vi "PLL.vi"(2 "Local Oscillator":waveform(dbl), 3 "Input Waveform":waveform(dbl)) -> (0 "Phase Difference":dbl)   [LabVIEW 2014]
uses:
  <vilib>/Analysis/NI_AALPro.lvlib
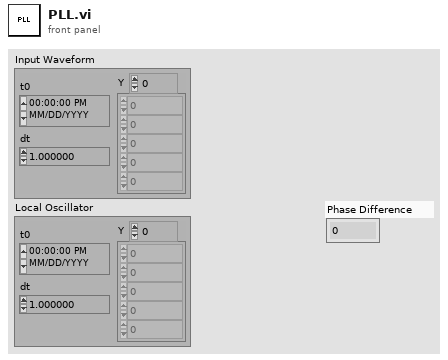
[diagram p1: front panel]
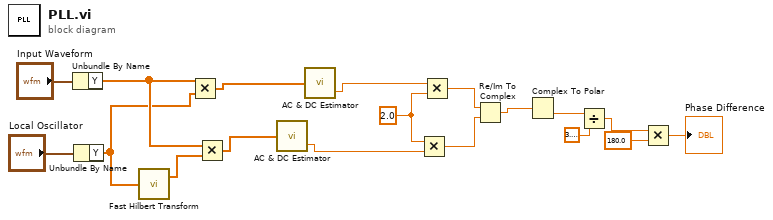
[diagram p0: block diagram]
diagram:
  w11 = 2.0 ("y")
  n1 = Unbundle By Name("Input Waveform") -> ("Y"=w18:dbl[])
  n2 = Unbundle By Name("Local Oscillator") -> ("Y"=w16:dbl[])
  n3 = call <vilib>:"Fast Hilbert Transform.vi"("X"=w16) -> ("Hilbert{X}"=w17:dbl[])  [unwired: 1 out]
  n4 = Multiply(x=w18, y=w16) -> (x*y=w14:dbl[])
  n5 = Multiply(x=w18, y=w17) -> (x*y=w15:dbl[])
  n6 = call <vilib>:"AC & DC Estimator.vi"("Signal (V)"=w15) -> ("DC estimate (V)"=w13:dbl)  [unwired: 1 out]
  n7 = call <vilib>:"AC & DC Estimator.vi"("Signal (V)"=w14) -> ("DC estimate (V)"=w12:dbl)  [unwired: 1 out]
  n8 = Multiply(x=w11, y=w13) -> (x*y=w9:dbl)
  n9 = Multiply(x=w12, y=w11) -> (x*y=w10:dbl)
  n10 = Re/Im To Complex(1:w9, 2:w10) -> (0:w8:cdb)
  n11 = Complex To Polar(r * e^(i*theta)=w8) -> (theta=w7:dbl)  [unwired: 1 out]
  n12 = Divide(x=w7, y=3.141592653589793) -> (x/y=w5:dbl)
  n13 = Multiply(x=w5, y=180.0) -> (x*y=→"Phase Difference":dbl)
